vi "SingleStripQuality.vi"(2 "R standard deviation":dbl format="%.2f", 3 "R mean":dbl format="%.2f", 4 "Thresholds":T1, 5 "Pinhole flag in":i32, 6 "Resistance Data":dbl, 7 "Capacitance Data":dbl) -> (0 "Defect Type":string, 1 "Defect Flag":i32)   [LabVIEW 2019]
panel:
  in  "Defect Code":i32
  # "Current [nA]:"
  # "Capacitance [pF]:"
  # "Resistance [MW]:"
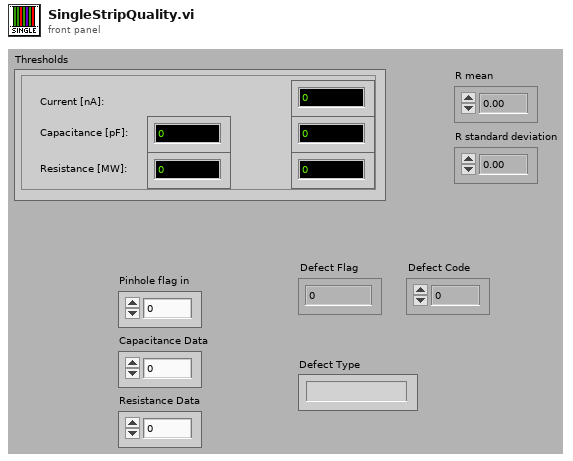
[diagram p1: front panel]
types:
  T1 = cluster{"Current [nA]":dbl, "Cap_Lo":dbl, "Cap_Hi":dbl, "Res_Hi":dbl, "Res_Lo":dbl}
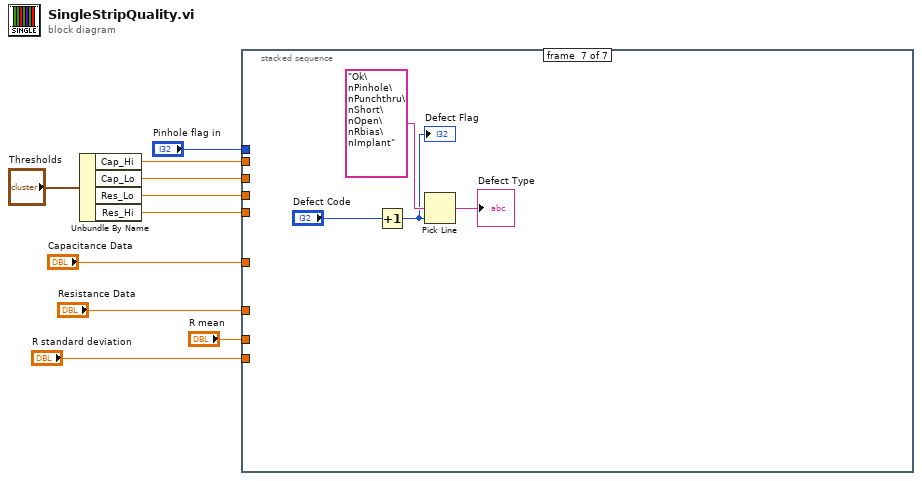
[diagram p0: block diagram]
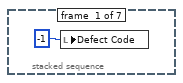
[diagram p2: hidden frame]
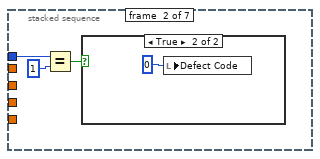
[diagram p3: hidden frame]
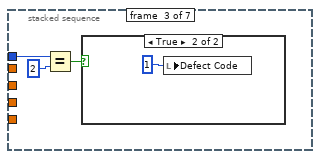
[diagram p5: hidden frame]
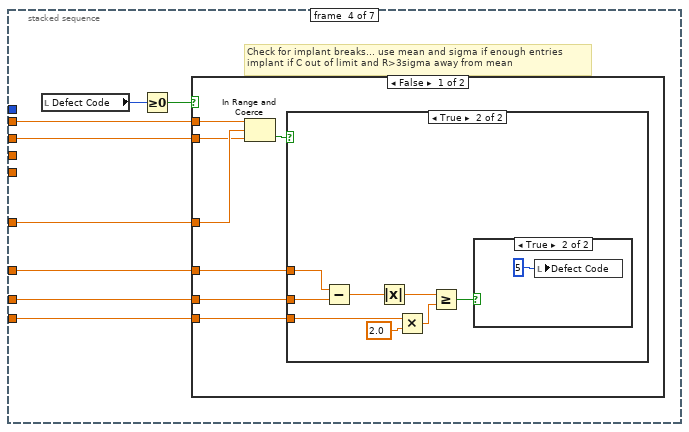
[diagram p7: hidden frame]
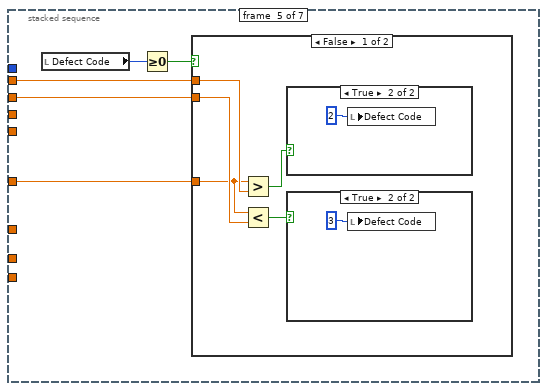
[diagram p11: hidden frame]
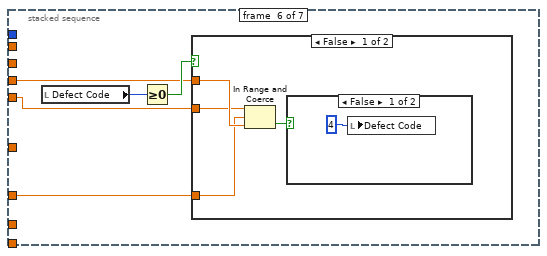
[diagram p15: hidden frame]
diagram:
  n1 = Unbundle By Name("Thresholds") -> ("Cap_Hi"=w10:dbl, "Cap_Lo"=w9:dbl, "Res_Lo"=w8:dbl, "Res_Hi"=w7:dbl)
  n2 = stacked-sequence {
    tunnel: w10 -> [_ _ _ w25 w46 _ _]
    tunnel: w9 -> [_ _ _ w24 w45 _ _]
    tunnel: w8 -> [_ _ _ _ _ w58 _]
    tunnel: w7 -> [_ _ _ _ _ w57 _]
    tunnel: "Pinhole flag in" -> [_ w13 w17 _ _ _ _]
    tunnel: "Capacitance Data" -> [_ _ _ w23 w44 _ _]
    tunnel: "Resistance Data" -> [_ _ _ w22 _ w56 _]
    tunnel: "R mean" -> [_ _ _ w21 _ _ _]
    tunnel: "R standard deviation" -> [_ _ _ w20 _ _ _]
    frame #0 {
      n3 = local write "Defect Code"(-1 ("Defect code")) -> ()
    }
    frame #1 {
      n4 = Equal?(x=w13, y=1) -> (x = y?=w14:bool)
      n5 = case shown="True" w14 {
        frame False {
        }
        frame True {
          n6 = local write "Defect Code"(0 ("Defect code")) -> ()
        }
      }
    }
    frame #2 {
      n7 = Equal?(x=w17, y=2) -> (x = y?=w18:bool)
      n8 = case shown="True" w18 {
        frame False {
        }
        frame True {
          n9 = local write "Defect Code"(1 ("Defect code")) -> ()
        }
      }
    }
    frame #3 {
      # "Check for implant breaks... use mean and sigma if enough entries\nimplant if C out of limit and R>3sigma away from mean"
      n10 = local read "Defect Code"() -> (w27:i32)
      n11 = Greater Or Equal To 0?(x=w27) -> (x >= 0?=w26:bool)
      n12 = case shown="False" w26 {
        tunnel: w23 -> [w34 _]
        tunnel: w25 -> [w33 _]
        tunnel: w24 -> [w32 _]
        tunnel: w22 -> [w30 _]
        tunnel: w21 -> [w29 _]
        tunnel: w20 -> [w28 _]
        frame False {
          n13 = In Range and Coerce(upper limit=w33, x=w34, lower limit=w32) -> (In Range?=w31:bool)  [unwired: 1 out]
          n14 = case shown="True" w31 {
            tunnel: w30 -> [_ w37]
            tunnel: w29 -> [_ w36]
            tunnel: w28 -> [_ w35]
            frame False {
            }
            frame True {
              n15 = Subtract(x=w37, y=w36) -> (x-y=w42:dbl)
              n16 = Absolute Value(x=w42) -> (abs(x)=w40:dbl)
              n17 = Multiply(x=w35, y=2.0) -> (x*y=w39:dbl)
              n18 = Greater Or Equal?(x=w40, y=w39) -> (x >= y?=w38:bool)
              n19 = case shown="True" w38 {
                frame False {
                }
                frame True {
                  n20 = local write "Defect Code"(5 ("Defect code")) -> ()
                }
              }
            }
          }
        }
        frame True {
        }
      }
    }
    frame #4 {
      n21 = local read "Defect Code"() -> (w48:i32)
      n22 = Greater Or Equal To 0?(x=w48) -> (x >= 0?=w47:bool)
      n23 = case shown="False" w47 {
        tunnel: w46 -> [w53 _]
        tunnel: w45 -> [w51 _]
        tunnel: w44 -> [w49 _]
        frame False {
          n24 = Greater?(x=w49, y=w53) -> (0:w52:bool)
          n25 = Less?(x=w49, y=w51) -> (x < y?=w50:bool)
          n26 = case shown="True" w52 {
            frame False {
            }
            frame True {
              n27 = local write "Defect Code"(2 ("Defect code")) -> ()
            }
          }
          n28 = case shown="True" w50 {
            frame False {
            }
            frame True {
              n29 = local write "Defect Code"(3 ("Defect code")) -> ()
            }
          }
        }
        frame True {
        }
      }
    }
    frame #5 {
      n30 = local read "Defect Code"() -> (w60:i32)
      n31 = Greater Or Equal To 0?(x=w60) -> (x >= 0?=w59:bool)
      n32 = case shown="False" w59 {
        tunnel: w58 -> [w64 _]
        tunnel: w57 -> [w63 _]
        tunnel: w56 -> [w61 _]
        frame False {
          n33 = In Range and Coerce(upper limit=w63, x=w61, lower limit=w64) -> (In Range?=w62:bool)  [unwired: 1 out]
          n34 = case shown="False" w62 {
            frame False {
              n35 = local write "Defect Code"(4 ("Defect code")) -> ()
            }
            frame True {
            }
          }
        }
        frame True {
        }
      }
    }
    frame #6 {
      n36 = Increment(x="Defect Code") -> (x+1=w67:i32)
      "Defect Flag" <- w67
      n37 = Pick Line(multi-line string="Ok\nPinhole\nPunchthru\nShort\nOpen\nRbias\nImplant", line index=w67) -> (output string=→"Defect Type":string)  [unwired: 1 in]
    }
  }
